vi "PWM_Threshold.vi"(1 "Input_PWM":dbl, 2 "Threshold":dbl) -> (0 "Trimmed_PWM":dbl)   [LabVIEW 2018]
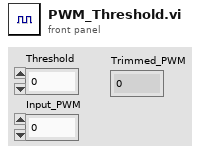
[diagram p1: front panel]
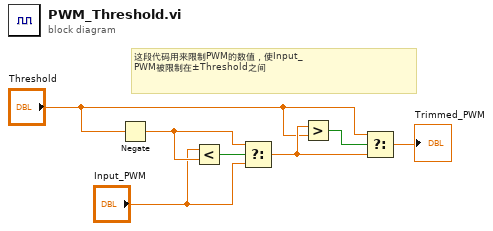
[diagram p0: block diagram]
diagram:
  # "这段代码用来限制PWM的数值，使Input_PWM被限制在±Threshold之间"
  n1 = Negate(x="Threshold") -> (-x=w4:dbl)
  n2 = Less?(x="Input_PWM", y=w4) -> (x < y?=w7:bool)
  n3 = Select(t=w4, s=w7, f="Input_PWM") -> (s? t:f=w5:dbl)
  n4 = Greater?(x=w5, y="Threshold") -> (0:w6:bool)
  n5 = Select(t="Threshold", s=w6, f=w5) -> (s? t:f=→"Trimmed_PWM":dbl)
